vi "Result.Measurement, Screen for Fail or Error.vi"(10 "Num":T1[](array[typedef]) {"Status" items=["LOG", "PASS", "FAIL", "ERROR"]}, 11 "ResultState In":T3={"State"=enum."Failing", "Code"=0, "Description"=""}) -> (3 "ResultState Out":T3={"State"=enum."Failing", "Code"=0, "Description"=""})   [LabVIEW 2018]
uses:
  <vilib>/KATE/SeqMgr/SeqMgr.Result Info.ctl
  <vilib>/KATE/SeqMgr/SeqMgr.Result State Enum.ctl
  Result.Measurement Item.ctl
  Result.Measurement and Attribute Item Status.ctl
  <vilib>/KATE/SeqMgr/SeqMgr.lvlib
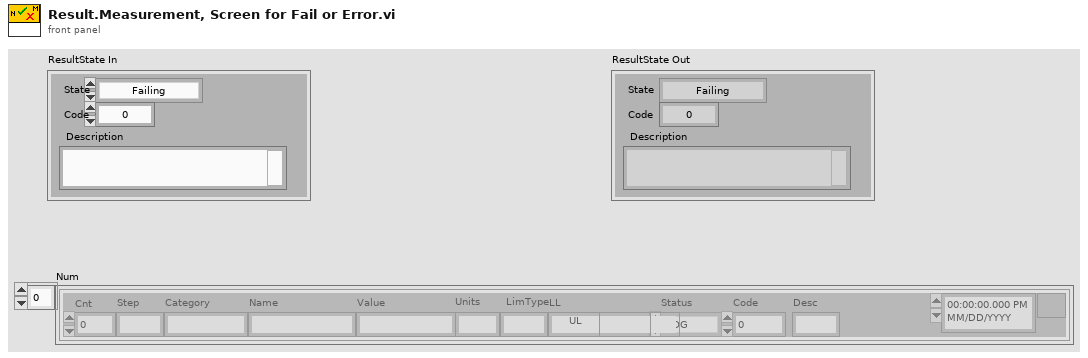
[diagram p1: front panel]
types:
  T1 = typedef "Result.Measurement Item.ctl" = cluster{"Cnt":i32, "Step":string, "Category":string, "Name":string, "Value":string, "Units":string, "LimType":string, "LL":string, "UL":string, "Status":T2, "Code":i32, "Desc":string, "Time":timestamp}
  T2 = typedef "Result.Measurement and Attribute Item Status.ctl" = i32
  T3 = typedef "KATE_Lib.lvlib/SeqMgr.lvlib/SeqMgr.Result Info.ctl" = cluster{"State":T4, "Code":i32, "Description":string}
  T4 = typedef "KATE_Lib.lvlib/SeqMgr.lvlib/SeqMgr.Result State Enum.ctl" = enum16{"None", "Passing", "Failing", "PASS", "FAIL", "ABORT", "ERROR"}
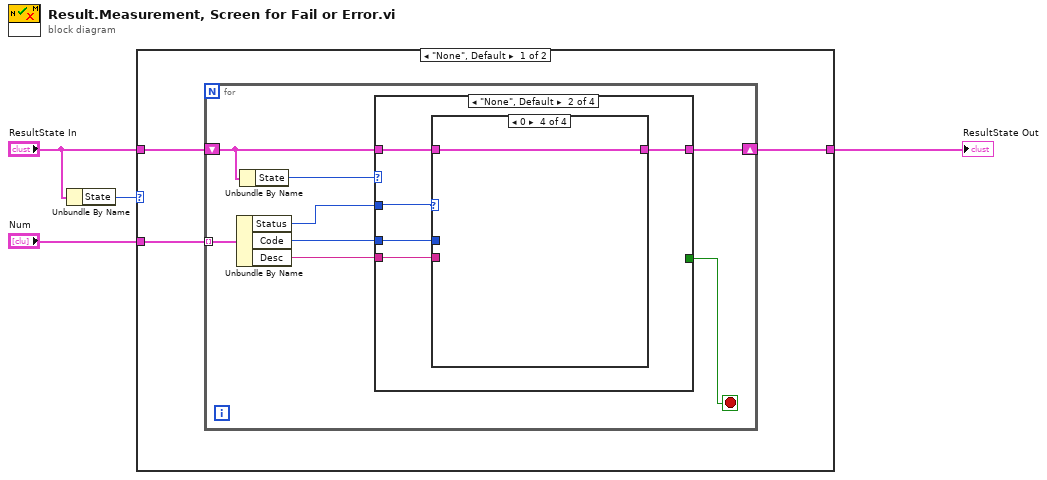
[diagram p0: block diagram]
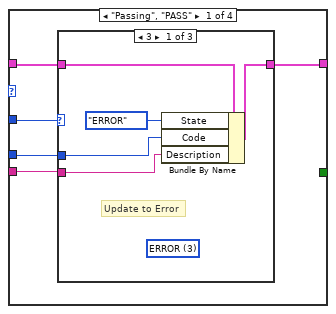
[diagram p2: hidden frame]
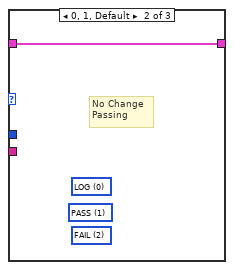
[diagram p3: hidden frame]
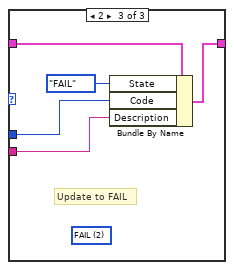
[diagram p4: hidden frame]
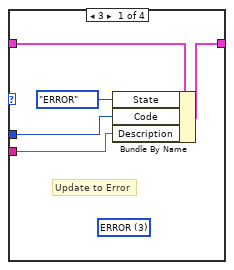
[diagram p5: hidden frame]
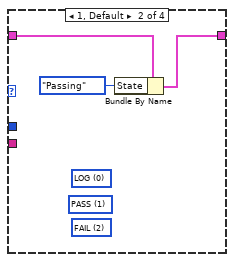
[diagram p6: hidden frame]
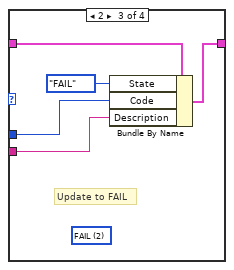
[diagram p7: hidden frame]
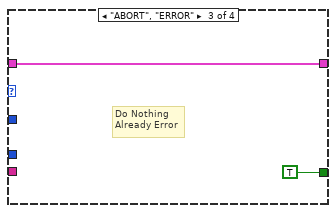
[diagram p8: hidden frame]
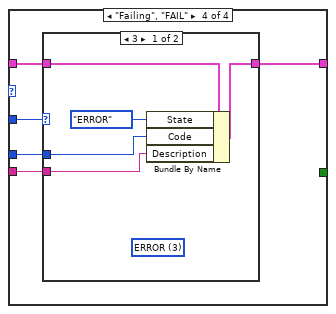
[diagram p9: hidden frame]
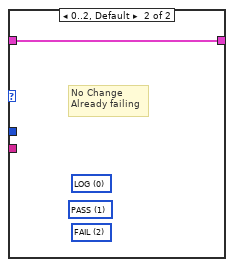
[diagram p10: hidden frame]
diagram:
  n1 = Unbundle By Name("ResultState In") -> ("State"=w3:T4)
  n2 = case shown="\"None\", Default" w3 {
    tunnel: "Num" -> [w7 _]
    tunnel: "ResultState In" -> [w6 w64]
    tunnel: [w5 w64] -> w1
    frame "None", Default {
      n3 = for {
        tunnel: w7 -> [w15] mode=indexing
        shift-right: [w9] -> w5
        shift-left: w6 -> [w13]
        stop <- w8 stop-if-true
        n4 = Unbundle By Name(w15) -> ("Status"=w12:T2, "Code"=w11:i32, "Desc"=w10:string)
        n5 = Unbundle By Name(w13) -> ("State"=w14:T4)
        n6 = case shown="\"None\", Default" w14 {
          tunnel: w13 -> [w20 w35 w51 w57]
          tunnel: [_ _ TRUE _] -> w8
          tunnel: [w16 w36 w51 w55] -> w9
          tunnel: w12 -> [w19 w34 _ w56]
          tunnel: w11 -> [w18 w33 _ w54]
          tunnel: w10 -> [w17 w32 _ w53]
          frame "Passing", "PASS" {
            n7 = case shown="3" w19 {
              tunnel: w20 -> [w25 w26 w30]
              tunnel: [w24 w26 w29] -> w16
              tunnel: w18 -> [w23 _ w28]
              tunnel: w17 -> [w22 _ w27]
              frame 3 {
                (unwired) T2 3 items=["LOG", "PASS", "FAIL", "ERROR"] ("Status")
                # "Update to Error"
                n8 = Bundle By Name(cluster=w25, "State"=SeqMgr.Result_State_Enum."ERROR", "Code"=w23, "Description"=w22) -> (w24:T3)
              }
              frame 0, 1, Default {
                (unwired) T2 2 items=["LOG", "PASS", "FAIL", "ERROR"] ("Status")
                (unwired) T2 1 items=["LOG", "PASS", "FAIL", "ERROR"] ("Status")
                (unwired) T2 0 items=["LOG", "PASS", "FAIL", "ERROR"] ("Status")
                # "No Change\nPassing"
              }
              frame 2 {
                (unwired) T2 2 items=["LOG", "PASS", "FAIL", "ERROR"] ("Status")
                # "Update to FAIL"
                n9 = Bundle By Name(cluster=w30, "State"=SeqMgr.Result_State_Enum."FAIL", "Code"=w28, "Description"=w27) -> (w29:T3)
              }
            }
          }
          frame "None", Default {
            n10 = case shown="0" w34 {
              tunnel: w35 -> [w41 w44 w48 w50]
              tunnel: [w40 w43 w47 w50] -> w36
              tunnel: w33 -> [w39 _ w46 _]
              tunnel: w32 -> [w38 _ w45 _]
              frame 3 {
                (unwired) T2 3 items=["LOG", "PASS", "FAIL", "ERROR"] ("Status")
                # "Update to Error"
                n11 = Bundle By Name(cluster=w41, "State"=SeqMgr.Result_State_Enum."ERROR", "Code"=w39, "Description"=w38) -> (w40:T3)
              }
              frame 1, Default {
                (unwired) T2 2 items=["LOG", "PASS", "FAIL", "ERROR"] ("Status")
                (unwired) T2 1 items=["LOG", "PASS", "FAIL", "ERROR"] ("Status")
                (unwired) T2 0 items=["LOG", "PASS", "FAIL", "ERROR"] ("Status")
                n12 = Bundle By Name(cluster=w44, "State"=SeqMgr.Result_State_Enum."Passing") -> (w43:T3)
              }
              frame 2 {
                (unwired) T2 2 items=["LOG", "PASS", "FAIL", "ERROR"] ("Status")
                # "Update to FAIL"
                n13 = Bundle By Name(cluster=w48, "State"=SeqMgr.Result_State_Enum."FAIL", "Code"=w46, "Description"=w45) -> (w47:T3)
              }
              frame 0 {
              }
            }
          }
          frame "ABORT", "ERROR" {
            # "Do Nothing\nAlready Error"
          }
          frame "Failing", "FAIL" {
            n14 = case shown="3" w56 {
              tunnel: w57 -> [w62 w63]
              tunnel: [w61 w63] -> w55
              tunnel: w54 -> [w60 _]
              tunnel: w53 -> [w59 _]
              frame 3 {
                (unwired) T2 3 items=["LOG", "PASS", "FAIL", "ERROR"] ("Status")
                n15 = Bundle By Name(cluster=w62, "State"=SeqMgr.Result_State_Enum."ERROR", "Code"=w60, "Description"=w59) -> (w61:T3)
              }
              frame 0..2, Default {
                (unwired) T2 2 items=["LOG", "PASS", "FAIL", "ERROR"] ("Status")
                (unwired) T2 1 items=["LOG", "PASS", "FAIL", "ERROR"] ("Status")
                (unwired) T2 0 items=["LOG", "PASS", "FAIL", "ERROR"] ("Status")
                # "No Change\nAlready failing"
              }
            }
          }
        }
      }
    }
    frame "ERROR" {
      # "Already at error - no change"
    }
  }
  "ResultState Out" <- w1
